vi "PH_SHS_Analysis.evt call Remove Tilt.vi"(0 "i ref in":refnum<vi>, 1 "Instance":string, 5 "error in (no error)":errorcluster) -> (14 "i ref out":refnum<vi>, 19 "error out":errorcluster)   [LabVIEW 2014, in "PH_SHS_Analysis.lvlib"]
doc: "This VI calls the event case \"RemoveTilt\" by a simple call."
uses:
  PH_SHS_Analysis.lvlib
  CSCore/BaseProcess/BaseProcess.lvlib
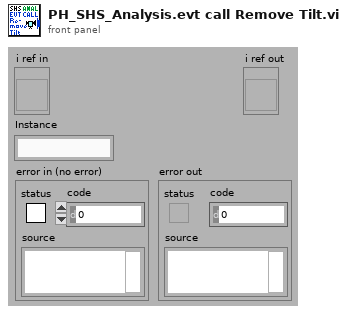
[diagram p1: front panel]
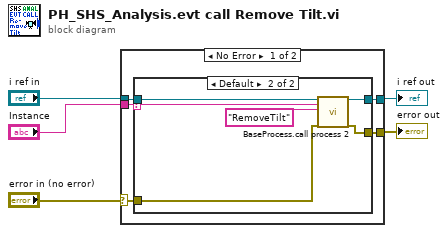
[diagram p0: block diagram]
diagram:
  n1 = case shown="No Error" "error in (no error)" {
    selector: "error in (no error)" -> [w7 w19]
    tunnel: [w10 w20] -> w2
    tunnel: [w9 w19] -> w1
    tunnel: "i ref in" -> [w8 w20]
    tunnel: "Instance" -> [w6 _]
    frame No Error {
      n2 = case shown="Default" w6 {
        selector: w6 -> [_ w13]
        tunnel: [w12 w17] -> w10
        tunnel: [w11 w16] -> w9
        tunnel: w8 -> [w12 w15]
        tunnel: w7 -> [w11 w14]
        frame "N/A" {
        }
        frame Default {
          n3 = call "BaseProcess.call process 2.vi"("i ref in"=w15, "Object"=w13, "Selector"="RemoveTilt", "error in (no error)"=w14) -> ("i ref out"=w17:refnum<vi>, "error out"=w16:errorcluster)  [unwired: 14 in]
        }
      }
    }
    frame Error {
    }
  }
  "i ref out" <- w2
  "error out" <- w1
